vi "set_libraryBlacklist_p.vi"(0 "MoAgSy_Host":refnum<class "MoAgSy_Host.lvclass">, 2 "Library Blacklist":string[](array[string]), 5 "error in (no error)":errorcluster) -> (14 "dup MoAgSy_Host":refnum<class "MoAgSy_Host.lvclass">, 19 "error out":errorcluster)   [LabVIEW 2009, in "MoAgSy.lvlib" / "MoAgSy_Host.lvclass"]
doc: "<B>protected</B> VI sets blacklisted libraries for mobile agent host class.\nIs called by public set library Blacklist VI\n\nF.Berck@gsi.de\nGSI Darmstadt 2009"
uses:
  MoAgSy_Host.lvclass
  MoAgSy_Host.lvclass/MoAgSy_Host.ctl
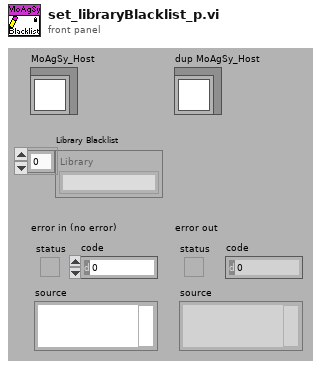
[diagram p1: front panel]
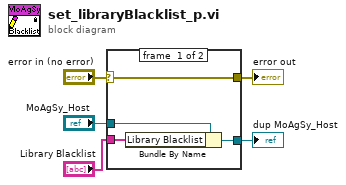
[diagram p0: block diagram]
diagram:
  n1 = case shown="No Error" "error in (no error)" {
    selector: "error in (no error)" -> [w9 w10]
    tunnel: [w9 w10] -> w4
    tunnel: [w7 w11] -> w2
    tunnel: "MoAgSy_Host" -> [w8 w11]
    tunnel: "Library Blacklist" -> [w6 _]
    frame #0 {
      n2 = Bundle By Name(cluster=w8, "Library Blacklist"=w6) -> (w7:refnum<class "MoAgSy_Host.lvclass">)
    }
    frame #1 {
    }
  }
  "error out" <- w4
  "dup MoAgSy_Host" <- w2
